vi "Input Control.vi"(5 "State":enum16{"Open", "Run", "End"}(ring)) -> (0 "Secondary Joystick":T2, 1 "Twist-handle Joystick":T3, 2 "Gamepad":T4)   [LabVIEW 2013]
doc: "This VI will initialize human interface devices for use with the robot. It is compatible with any device provided your PC has the proper drivers installed. It has been specifically written to function with either a gamepad or dual joysticks, but will function with any devices. It can get values for up to 6 axes and 12 buttons per device, and if the devices used are one of the kinds of devices that this VI was specifically written for, you will have the added bonus of prenamed outputs! For two input devices to be controlled simultaniously, use the \"Joysticks\" device input. If you only need one, esp. if the device is a gamepad, use the \"Controller\" device input setting. Two gamepads CAN be operated simultaniously by this VI, but you will not have the niceties of axes pregrouped into their respective joysticks.\n\nThe following inputs are required:\n State must be \"Open\" when initializing, \"Run\" when output values are necessary, and \"End\" at the end of your program.\n Device must be specified as described above.\n\nThe following outputs are required when the Device input is set to \"Joysticks\" to recieve data:\n Joystick 1 must be wired to an \"Unbundle\" block followed by two more \"Unbundle\" blocks to get the individual values. Use \"Unbundle By Name\" to use the names associated with the outputs.\n Joystick 2 must be wired to an \"Unbundle\" block followed by two more \"Unbundle\" blocks to get the individual values. Use \"Unbundle By Name\" to use the names associated with the outputs.\n\nThe following outputs are required when the Device input is set to \"Controller\" to recieve data:\n Controller must be wired to an \"Unbundle\" block followed by another \"Unbundle\" block for each data wire. The \"Axes\" subcluster contains two more clusters which contain the joystick values. \"Unbundle\" them to get values for the joysticks. The triggers (axis 3) are not contained within a subcluster of \"Axes\" and their value is available immediately."
uses:
  <vilib>/Rock Robotics/WPI/Joystick/WPI_JoystickButtonState.ctl
  <vilib>/Rock Robotics/WPI/Joystick/WPI_JoystickDeviceEnum.ctl
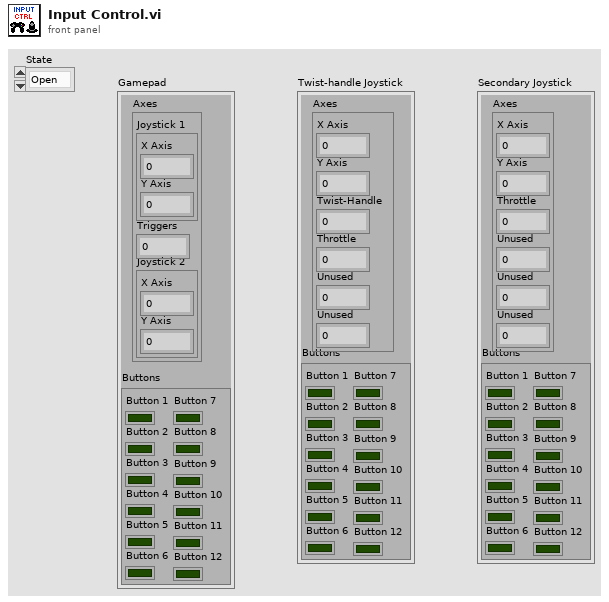
[diagram p1: front panel]
types:
  T1 = typedef "WPI_JoystickButtonState.ctl" = cluster{"Button 1":bool, "Button 2":bool, "Button 3":bool, "Button 4":bool, "Button 5":bool, "Button 6":bool, "Button 7":bool, "Button 8":bool, "Button 9":bool, "Button 10":bool, "Button 11":bool, "Button 12":bool}
  T2 = cluster{"Axes":cluster{"X Axis":dbl, "Y Axis":dbl, "Throttle":dbl, "Unused":dbl, "Unused":dbl, "Unused":dbl}, "Buttons":T1}
  T3 = cluster{"Axes":cluster{"X Axis":dbl, "Y Axis":dbl, "Twist-Handle":dbl, "Throttle":dbl, "Unused":dbl, "Unused":dbl}, "Buttons":T1}
  T4 = cluster{"Axes":cluster{"Joystick 1":cluster{"X Axis":dbl, "Y Axis":dbl}, "Triggers":dbl, "Joystick 2":cluster{"X Axis":dbl, "Y Axis":dbl}}, "Buttons":T1}
  T5 = typedef "WPI_JoystickDeviceEnum.ctl" = enum16{"USB 1", "USB 2", "USB 3", "USB 4", "Kinect 1", "Kinect 2"}
  T6 = typedef "WPI_JoystickDevRef.ctl" = cluster{"Device":T5}
  T7 = cluster{"axis 1 (x)":dbl, "axis 2 (y)":dbl, "axis 3 (throttle)":dbl, "axis 4":dbl, "axis 5":dbl, "axis 6":dbl}
  T8 = cluster{"Axes":cluster{"axis 1 (x)":dbl, "axis 2 (y)":dbl, "axis 3 (throttle)":dbl, "axis 4":dbl, "axis 5":dbl, "axis 6":dbl}, "Buttons":T1}
  T9 = cluster{"Output 5":dbl, "Output 6":dbl, "Output 7":dbl, "axis 4":dbl, "axis 5":dbl, "axis 6":dbl}
  T10 = cluster{cluster{"Output 1":dbl, "Output 2":dbl}, "axis 3 (throttle)":dbl, cluster{"Output 3":dbl, "Output 4":dbl}}
  T11 = cluster{cluster{"Output 5":dbl, "Output 6":dbl, "Output 7":dbl, "axis 4":dbl, "axis 5":dbl, "axis 6":dbl}, "Buttons":T1}
  T12 = cluster{cluster{cluster{"Output 1":dbl, "Output 2":dbl}, "axis 3 (throttle)":dbl, cluster{"Output 3":dbl, "Output 4":dbl}}, "Buttons":T1}
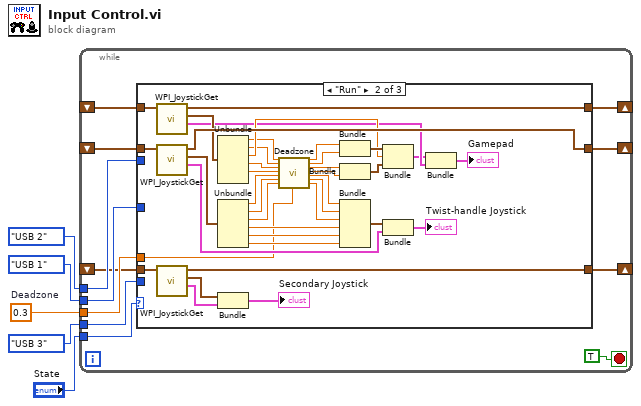
[diagram p0: block diagram]
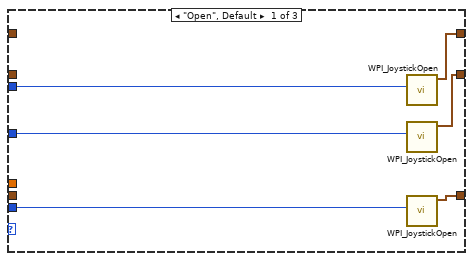
[diagram p2: hidden frame]
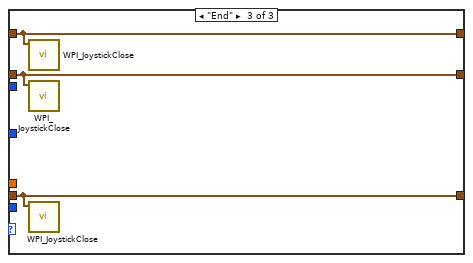
[diagram p3: hidden frame]
diagram:
  w1 = 0.3  # Deadzone
  n1 = while {
    tunnel: "State" -> [w17]
    tunnel: WPI_JoystickDeviceEnum."USB 2" ("Controller") -> [w16]
    tunnel: WPI_JoystickDeviceEnum."USB 1" ("Controller") -> [w15]
    tunnel: WPI_JoystickDeviceEnum."USB 3" ("Controller") -> [w14]
    tunnel: w1 -> [w13]
    shift-right: [w11] -> _
    shift-left: _ -> [w8]
    shift-right: [w10] -> _
    shift-left: _ -> [w7]
    shift-right: [w9] -> _
    shift-left: _ -> [w6]
    stop <- TRUE stop-if-true
    n2 = case shown="\"Run\"" w17 {
      tunnel: w16 -> [w23 _ _]
      tunnel: [w22 w59 w64] -> w11
      tunnel: [w21 w60 w63] -> w10
      tunnel: w15 -> [w20 _ _]
      tunnel: w14 -> [w19 _ _]
      tunnel: [w18 w61 w62] -> w9
      tunnel: w13 -> [_ w27 _]
      tunnel: w8 -> [_ w26 w64]
      tunnel: w7 -> [_ w25 w63]
      tunnel: w6 -> [_ w24 w62]
      frame "Open", Default {
        n3 = call <vilib>:"WPI_JoystickOpen.vi"("JoystickDevice"=w23) -> ("JoystickDevRef"=w22:T6)  [unwired: 10 in]
        n4 = call <vilib>:"WPI_JoystickOpen.vi"("JoystickDevice"=w20) -> ("JoystickDevRef"=w21:T6)  [unwired: 10 in]
        n5 = call <vilib>:"WPI_JoystickOpen.vi"("JoystickDevice"=w19) -> ("JoystickDevRef"=w18:T6)  [unwired: 10 in]
      }
      frame "Run" {
        n6 = call <vilib>:"WPI_JoystickGet.vi"("JoystickDevRef"=w26) -> ("Buttons"=w54:T1, "Axes"=w58:T7, "JoystickDevRef"=w59:T6)  [unwired: 4 in]
        n7 = call <vilib>:"WPI_JoystickGet.vi"("JoystickDevRef"=w25) -> ("Buttons"=w50:T1, "Axes"=w51:T7, "JoystickDevRef"=w60:T6)  [unwired: 4 in]
        n8 = call <vilib>:"WPI_JoystickGet.vi"("JoystickDevRef"=w24) -> ("Buttons"=w47:T1, "Axes"=w48:T7, "JoystickDevRef"=w61:T6)  [unwired: 4 in]
        n9 = Unbundle(w58) -> ("axis 1 (x)"=w45:dbl, "axis 2 (y)"=w44:dbl, "axis 3 (throttle)"=w56:dbl, "axis 4"=w43:dbl, "axis 5"=w42:dbl)  [unwired: 1 out]
        n10 = Unbundle(w51) -> ("axis 1 (x)"=w37:dbl, "axis 2 (y)"=w36:dbl, "axis 3 (throttle)"=w35:dbl, "axis 4"=w30:dbl, "axis 5"=w29:dbl, "axis 6"=w28:dbl)
        n11 = Bundle("Axes"=w48, "Buttons"=w47) -> (→"Secondary Joystick":T8)  [unwired: 1 in]
        n12 = call "Deadzone.vi"("Input 1"=w45, "Input 2"=w44, "Input 3"=w43, "Input 4"=w42, "Input 5"=w37, "Input 6"=w36, "Input 7"=w35, "Deadzone"=w27) -> ("Output 1"=w41:dbl, "Output 2"=w40:dbl, "Output 3"=w39:dbl, "Output 4"=w38:dbl, "Output 5"=w33:dbl, "Output 6"=w31:dbl, "Output 7"=w32:dbl)  [unwired: 12 in, 1 out]
        n13 = Bundle("Output 1"=w41, "Output 2"=w40) -> (w57:cluster{"Output 1":dbl, "Output 2":dbl})  [unwired: 1 in]
        n14 = Bundle("Output 3"=w39, "Output 4"=w38) -> (w55:cluster{"Output 3":dbl, "Output 4":dbl})  [unwired: 1 in]
        n15 = Bundle("Output 5"=w33, "Output 6"=w31, "Output 7"=w32, "axis 4"=w30, "axis 5"=w29, "axis 6"=w28) -> (w34:T9)  [unwired: 1 in]
        n16 = Bundle(w57, "axis 3 (throttle)"=w56, w55) -> (w53:T10)  [unwired: 1 in]
        n17 = Bundle(w34, "Buttons"=w50) -> (→"Twist-handle Joystick":T11)  [unwired: 1 in]
        n18 = Bundle(w53, "Buttons"=w54) -> (→"Gamepad":T12)  [unwired: 1 in]
      }
      frame "End" {
        n19 = call <vilib>:"WPI_JoystickClose.vi"("JoystickDevRef"=w64) -> ()  [unwired: 11 in]
        n20 = call <vilib>:"WPI_JoystickClose.vi"("JoystickDevRef"=w63) -> ()  [unwired: 11 in]
        n21 = call <vilib>:"WPI_JoystickClose.vi"("JoystickDevRef"=w62) -> ()  [unwired: 11 in]
      }
    }
  }
